vi "Shutdown KnownHosts.vi"(8 "Error In":errorcluster, 10 "Handle":u64, 11 "Session In":refnum<class "Session.lvclass">) -> (0 "Error Out":errorcluster, 3 "Session Out":refnum<class "Session.lvclass">)   [LabVIEW 2017, in "LabSSH2.lvlib" / "Session.lvclass"]
uses:
  Session.lvclass
  Session.lvclass/Session.ctl
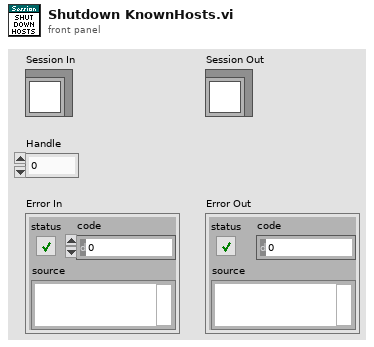
[diagram p1: front panel]
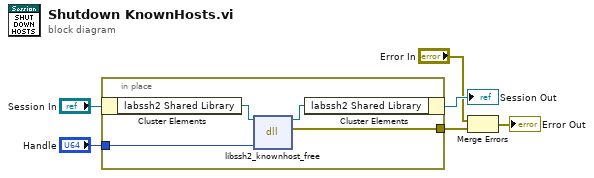
[diagram p0: block diagram]
diagram:
  n1 = in-place {
    in-place-border: [w8] -> w6
    in-place-border: "Handle" -> [w7]
    n2 = in-place-cluster #1("Session In") -> ("labssh2 Shared Library"=w10:path)
    n3 = dll-call lib="D:/Users/cfield/Code/Field R&D Services/SSH/LabSSH2/LabVIEW/trunk/src/LabSSH2/Private/labssh2.*" fn="libssh2_knownhost_free"(path in=w10, "hosts"=w7) -> (path out=w9:path, error out=w8:errorcluster)  [unwired: 4 in]
    n4 = in-place-cluster #1("labssh2 Shared Library"=w9) -> (→"Session Out":refnum<class "Session.lvclass">)
  }
  n5 = Merge Errors("Error In", w6) -> (→"Error Out":errorcluster)
